vi "PicoScope3000aAdvancedTriggerSettings.vi"(0 "error in":errorcluster, 1 "handle in":i16, 3 "Trigger Conditions":T6 {"Condition Logic" items=["AND", "OR", "XOR"]}, 4 "Trigger Delay":u32, 5 "Auto Trigger (ms)":i32=1000, 6 "Channel A Trigger Properties":T3={"thresholdUpper"=0, "thresholdUpperHysteresis"=5, "thresholdLower"=0, "thresholdLowerHysteresis"=5, "Threshold Mode"=0, "Direction"=2, "Available"=FALSE} {"Direction" items=["Above / Inside", "Below / Outside", "Rising / Enter", "Falling / Exit", "Rising or Falling / Enter or Exit", "Above Lower", "Below Lower", "Rising Lower", "Falling Lower", "Positive Runt", "Negative Runt"]; "Threshold Mode" items=["Level", "Window"]}, 7 "Channel D Trigger Properties":T3={"thresholdUpper"=0, "thresholdUpperHysteresis"=0, "thresholdLower"=0, "thresholdLowerHysteresis"=0, "Threshold Mode"=0, "Direction"=2, "Available"=FALSE} {"Direction" items=["Above / Inside", "Below / Outside", "Rising / Enter", "Falling / Exit", "Rising or Falling / Enter or Exit", "Above Lower", "Below Lower", "Rising Lower", "Falling Lower", "Positive Runt", "Negative Runt"]; "Threshold Mode" items=["Level", "Window"]}, 8 "Channel B Trigger Properties":T3={"thresholdUpper"=0, "thresholdUpperHysteresis"=0, "thresholdLower"=0, "thresholdLowerHysteresis"=0, "Threshold Mode"=0, "Direction"=2, "Available"=FALSE} {"Direction" items=["Above / Inside", "Below / Outside", "Rising / Enter", "Falling / Exit", "Rising or Falling / Enter or Exit", "Above Lower", "Below Lower", "Rising Lower", "Falling Lower", "Positive Runt", "Negative Runt"]; "Threshold Mode" items=["Level", "Window"]}, 10 "Digital Port  0":T2 {"Direction Channel 7" items=["Don't Care", "Low", "High", "Rising", "Falling"]; "Direction Channel 6" items=["Don't Care", "Low", "High", "Rising", "Falling"]; "Direction Channel 5" items=["Don't Care", "Low", "High", "Rising", "Falling"]; "Direction Channel 4" items=["Don't Care", "Low", "High", "Rising", "Falling"]; "Direction Channel 3" items=["Don't Care", "Low", "High", "Rising", "Falling"]; "Direction Channel 2" items=["Don't Care", "Low", "High", "Rising", "Falling"]; "Direction Channel 1" items=["Don't Care", "Low", "High", "Rising", "Falling"]; "Direction Channel 0" items=["Don't Care", "Low", "High", "Rising", "Falling"]}, 11 "Ext. Trigger Properties":T3={"thresholdUpper"=0, "thresholdUpperHysteresis"=0, "thresholdLower"=0, "thresholdLowerHysteresis"=0, "Threshold Mode"=0, "Direction"=2, "Available"=FALSE} {"Direction" items=["Above / Inside", "Below / Outside", "Rising / Enter", "Falling / Exit", "Rising or Falling / Enter or Exit", "Above Lower", "Below Lower", "Rising Lower", "Falling Lower", "Positive Runt", "Negative Runt"]; "Threshold Mode" items=["Level", "Window"]}, 12 "Digital Port  1":T1 {"Direction Channel 15" items=["Don't Care", "Low", "High", "Rising", "Falling"]; "Direction Channel 14" items=["Don't Care", "Low", "High", "Rising", "Falling"]; "Direction Channel 13" items=["Don't Care", "Low", "High", "Rising", "Falling"]; "Direction Channel 12" items=["Don't Care", "Low", "High", "Rising", "Falling"]; "Direction Channel 11" items=["Don't Care", "Low", "High", "Rising", "Falling"]; "Direction Channel 10" items=["Don't Care", "Low", "High", "Rising", "Falling"]; "Direction Channel 9" items=["Don't Care", "Low", "High", "Rising", "Falling"]; "Direction Channel 8" items=["Don't Care", "Low", "High", "Rising", "Falling"]}, 13 "Aux. Trigger Properties":T3={"thresholdUpper"=0, "thresholdUpperHysteresis"=0, "thresholdLower"=0, "thresholdLowerHysteresis"=0, "Threshold Mode"=0, "Direction"=2, "Available"=FALSE} {"Direction" items=["Above / Inside", "Below / Outside", "Rising / Enter", "Falling / Exit", "Rising or Falling / Enter or Exit", "Above Lower", "Below Lower", "Rising Lower", "Falling Lower", "Positive Runt", "Negative Runt"]; "Threshold Mode" items=["Level", "Window"]}, 16 "Channel C Trigger Properties":T3={"thresholdUpper"=0, "thresholdUpperHysteresis"=0, "thresholdLower"=0, "thresholdLowerHysteresis"=0, "Threshold Mode"=0, "Direction"=2, "Available"=FALSE} {"Direction" items=["Above / Inside", "Below / Outside", "Rising / Enter", "Falling / Exit", "Rising or Falling / Enter or Exit", "Above Lower", "Below Lower", "Rising Lower", "Falling Lower", "Positive Runt", "Negative Runt"]; "Threshold Mode" items=["Level", "Window"]}, 18 "Pulse Width Qualifier Conditions":T5 {"Condition Logic" items=["AND", "OR", "XOR"]}, 19 "Pulse Width Qualifier Settings":T4={"Direction"=2, "Lower Limit"=0, "Upper Limit"=0, "Pulse Width Type"=0} {"Pulse Width Type" items=["None", "Less Than", "Greater Than", "In Range", "Out of Range"]; "Direction" items=["Rising"=2, "Falling"=3]}) -> (14 "error out":errorcluster, 15 "handle out":i16)   [LabVIEW 2010]
doc: "This VI is an interface for the advanced trigger features of the oscilloscope (a simple trigger can be set using PicoScope3000aSettings.vi, in which case it is not necessary to use this VI)."
uses:
  ps3000a.dll
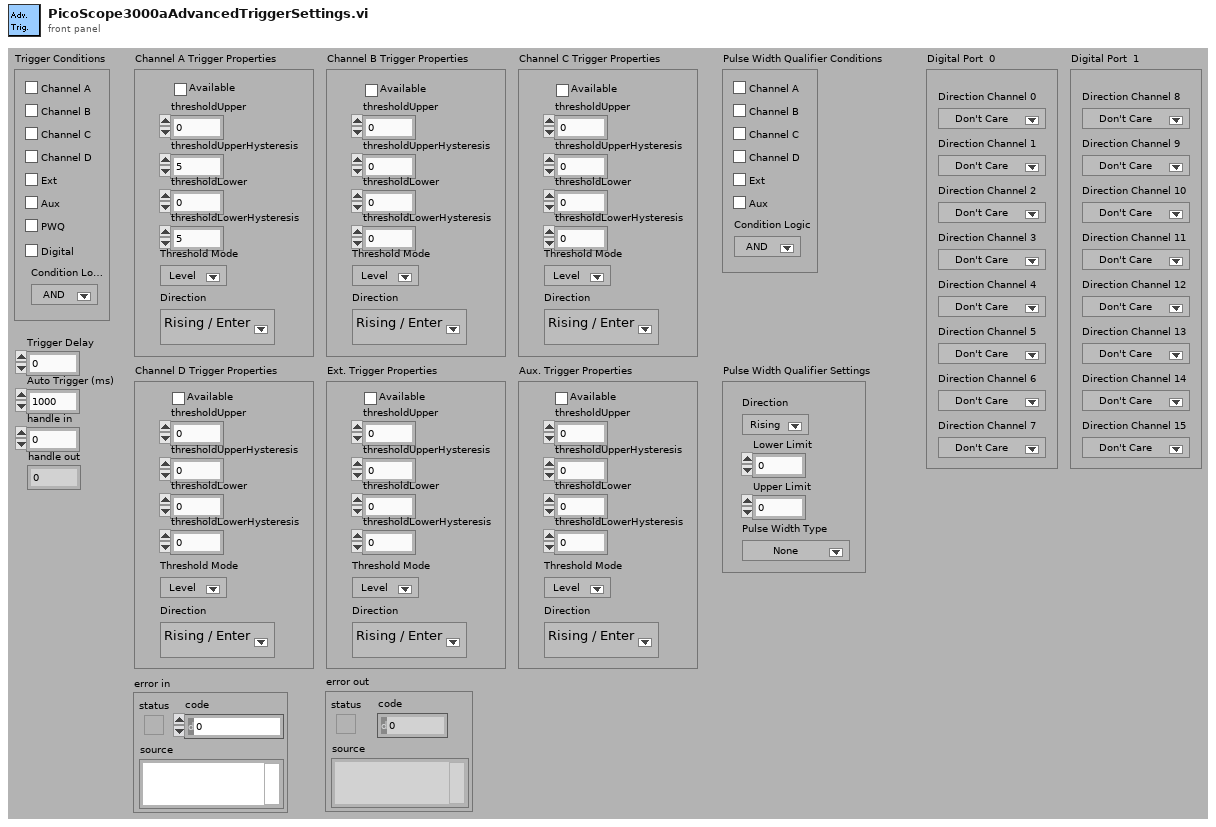
[diagram p1: front panel]
types:
  T1 = cluster{"Direction Channel 8":u16, "Direction Channel 9":u16, "Direction Channel 10":u16, "Direction Channel 11":u16, "Direction Channel 12":u16, "Direction Channel 13":u16, "Direction Channel 14":u16, "Direction Channel 15":u16}
  T2 = cluster{"Direction Channel 0":u16, "Direction Channel 1":u16, "Direction Channel 2":u16, "Direction Channel 3":u16, "Direction Channel 4":u16, "Direction Channel 5":u16, "Direction Channel 6":u16, "Direction Channel 7":u16}
  T3 = cluster{"thresholdUpper":i16, "thresholdUpperHysteresis":u16, "thresholdLower":i16, "thresholdLowerHysteresis":u16, "Threshold Mode":i32, "Direction":i32, "Available":bool}
  T4 = cluster{"Direction":u32, "Lower Limit":u32, "Upper Limit":u32, "Pulse Width Type":u32}
  T5 = cluster{"Channel A":bool, "Channel B":bool, "Channel C":bool, "Channel D":bool, "Aux":bool, "Condition Logic":u16, "Ext":bool}
  T6 = cluster{"Channel A":bool, "Channel B":bool, "Channel C":bool, "Channel D":bool, "Aux":bool, "PWQ":bool, "Condition Logic":u16, "Ext":bool, "Digital":bool}
  T7 = cluster{"thresholdUpper":i16, "thresholdUpperHysteresis":u16, "thresholdLower":i16, "thresholdLowerHysteresis":u16, "Threshold Mode":i32, "Direction":i32, "Available":bool}[]
  T8 = cluster{"[0]":u32, "[1]":u32, "[2]":u32, "[3]":u32, "[4]":u32, "[5]":u32, "[6]":u32, "[7]":u32, "[8]":u32}
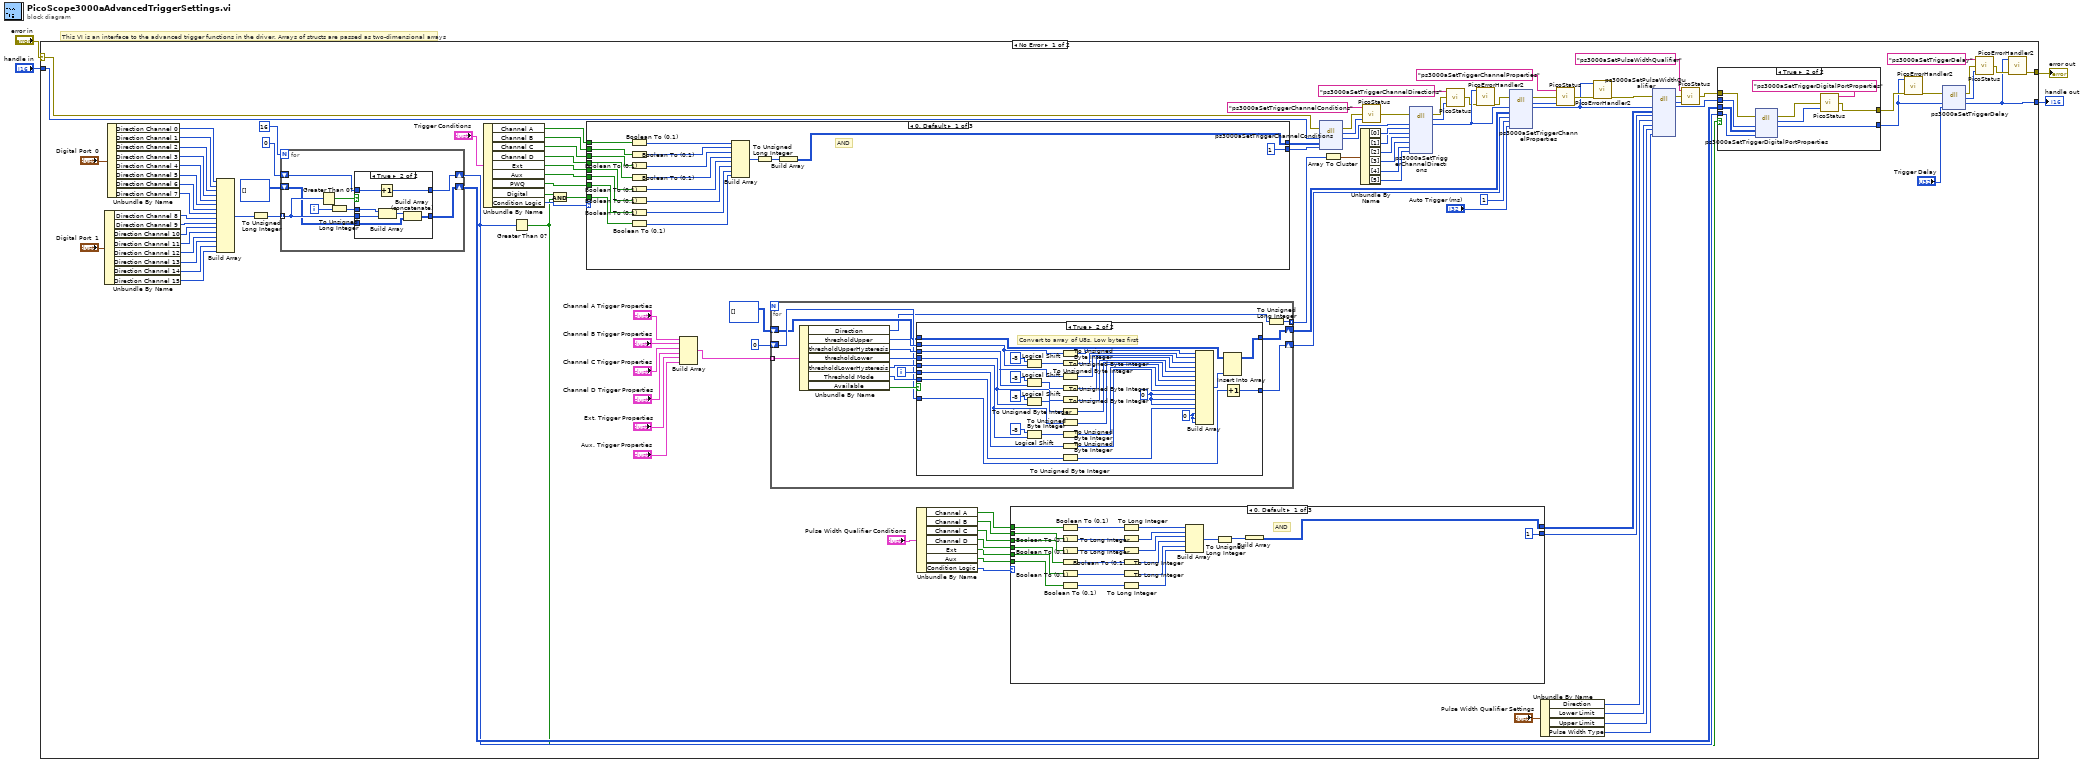
[diagram p0: block diagram]
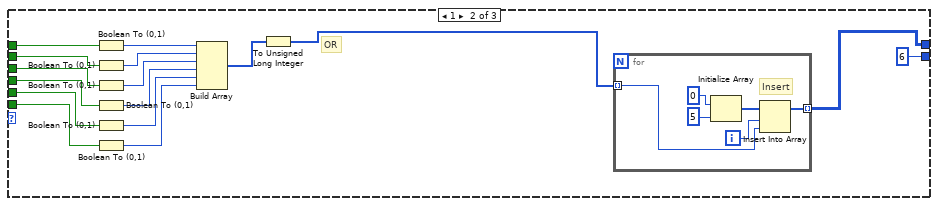
[diagram p4: hidden frame]
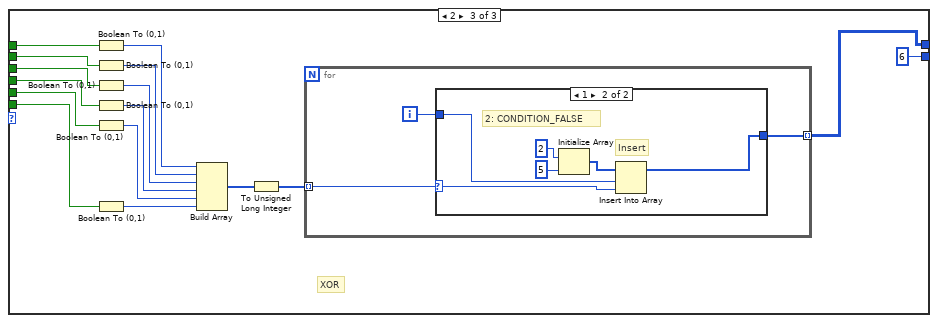
[diagram p5: hidden frame]
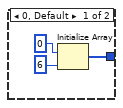
[diagram p6: hidden frame]
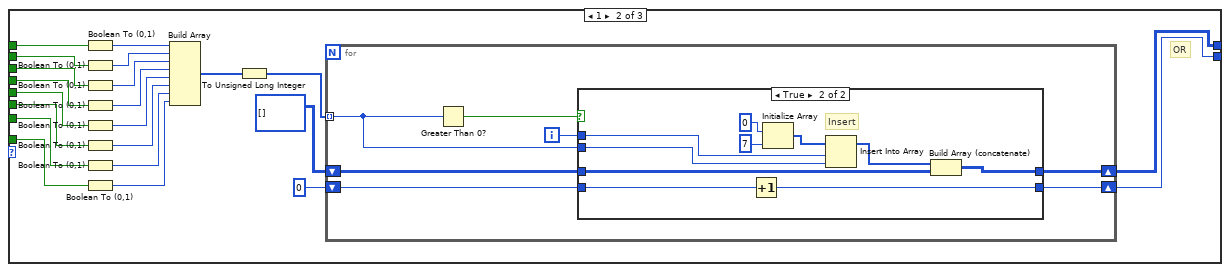
[diagram p8: hidden frame]
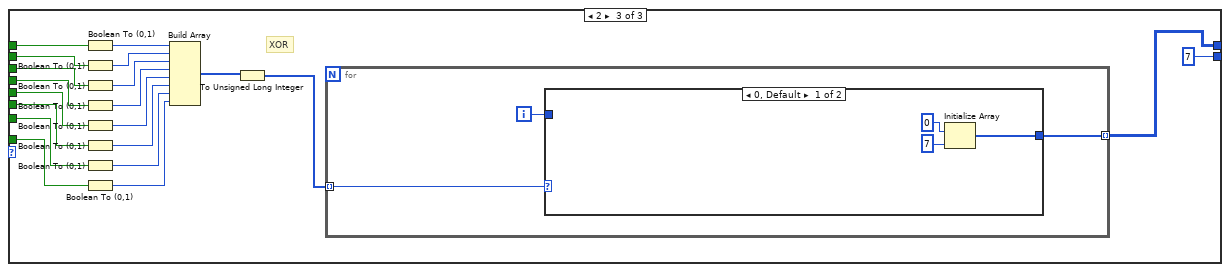
[diagram p10: hidden frame]
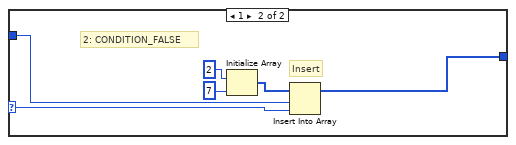
[diagram p11: hidden frame]
diagram:
  # "This VI is an interface to the advanced trigger functions in the driver. Arrays of structs are passed as two-dimensional arrays"
  n1 = case shown="No Error" "error in" {
    selector: "error in" -> [w73 w354]
    tunnel: "handle in" -> [w77 w355]
    tunnel: [w13 w355] -> w2
    tunnel: [w14 w354] -> w1
    frame No Error {
      n2 = Unbundle By Name("Digital Port  1") -> ("Direction Channel 8"=w38:u16, "Direction Channel 9"=w37:u16, "Direction Channel 10"=w36:u16, "Direction Channel 11"=w35:u16, "Direction Channel 12"=w34:u16, "Direction Channel 13"=w33:u16, "Direction Channel 14"=w32:u16, "Direction Channel 15"=w31:u16)
      n3 = Unbundle By Name("Digital Port  0") -> ("Direction Channel 0"=w50:u16, "Direction Channel 1"=w49:u16, "Direction Channel 2"=w48:u16, "Direction Channel 3"=w47:u16, "Direction Channel 4"=w46:u16, "Direction Channel 5"=w45:u16, "Direction Channel 6"=w44:u16, "Direction Channel 7"=w43:u16)
      n4 = Build Array(w50, w49, w48, w47, w46, w45, w44, w43, w38, w37, w36, w35, w34, w33, w32, w31) -> (w5:u16[])
      n5 = To Unsigned Long Integer(number=w5) -> (unsigned 32bit integer=w6:u32[])
      n6 = for {
        N: 16 -> [_]
        tunnel: w6 -> [w131] mode=indexing
        shift-right: [w130] -> w26
        shift-left: u32[][] [] -> [w129]
        shift-right: [w128] -> w23
        shift-left: i16 0 -> [w127]
        i -> [w125]
        n7 = Greater Than 0?(x=w131) -> (x > 0?=w132:bool)
        n8 = To Unsigned Long Integer(number=w125) -> (unsigned 32bit integer=w126:u32)
        n9 = case shown="True" w132 {
          tunnel: w126 -> [_ w141]
          tunnel: w131 -> [_ w140]
          tunnel: [w134 w138] -> w130
          tunnel: w129 -> [w134 w137]
          tunnel: [w133 w136] -> w128
          tunnel: w127 -> [w133 w135]
          frame False {
          }
          frame True {
            n10 = Increment(x=w135) -> (x+1=w136:i16)
            n11 = Build Array(w141, w140) -> (w139:u32[])
            n12 = Build Array (concatenate)(w139, w137) -> (w138:u32[][])
          }
        }
      }
      n13 = Unbundle By Name("Trigger Conditions") -> ("Channel A"=w57:bool, "Channel B"=w56:bool, "Channel C"=w55:bool, "Channel D"=w54:bool, "Ext"=w53:bool, "Aux"=w52:bool, "PWQ"=w51:bool, "Digital"=w25:bool, "Condition Logic"=w58:u16)
      n14 = Greater Than 0?(x=w23) -> (x > 0?=w22:bool)
      n15 = And(x=w25, y=w22) -> (x .and. y?=w24:bool)
      n16 = case shown="0, Default" w58 {
        tunnel: [w280 w295 w334] -> w110
        tunnel: [i16 1 w293 i16 7] -> w109
        tunnel: w57 -> [w278 w290 w331]
        tunnel: w56 -> [w277 w289 w330]
        tunnel: w55 -> [w276 w288 w329]
        tunnel: w54 -> [w275 w287 w328]
        tunnel: w53 -> [w274 w286 w327]
        tunnel: w52 -> [w273 w285 w326]
        tunnel: w51 -> [w272 w284 w325]
        tunnel: w24 -> [w271 w283 w324]
        frame 0, Default {
          # "AND"
          n17 = Boolean To (0,1)(Boolean=w278) -> (0, 1=w270:i16)
          n18 = Boolean To (0,1)(Boolean=w277) -> (0, 1=w269:i16)
          n19 = Boolean To (0,1)(Boolean=w276) -> (0, 1=w263:i16)
          n20 = Boolean To (0,1)(Boolean=w275) -> (0, 1=w264:i16)
          n21 = Boolean To (0,1)(Boolean=w274) -> (0, 1=w265:i16)
          n22 = Boolean To (0,1)(Boolean=w273) -> (0, 1=w266:i16)
          n23 = Boolean To (0,1)(Boolean=w272) -> (0, 1=w267:i16)
          n24 = Boolean To (0,1)(Boolean=w271) -> (0, 1=w268:i16)
          n25 = Build Array(w270, w269, w263, w264, w265, w266, w267, w268) -> (w262:i16[])
          n26 = To Unsigned Long Integer(number=w262) -> (unsigned 32bit integer=w261:u32[])
          n27 = Build Array(w261) -> (w280:u32[][])
        }
        frame 1 {
          # "OR"
          n28 = Boolean To (0,1)(Boolean=w290) -> (0, 1=w296:i16)
          n29 = Boolean To (0,1)(Boolean=w289) -> (0, 1=w297:i16)
          n30 = Boolean To (0,1)(Boolean=w288) -> (0, 1=w298:i16)
          n31 = Boolean To (0,1)(Boolean=w287) -> (0, 1=w299:i16)
          n32 = Boolean To (0,1)(Boolean=w286) -> (0, 1=w300:i16)
          n33 = Boolean To (0,1)(Boolean=w285) -> (0, 1=w301:i16)
          n34 = Boolean To (0,1)(Boolean=w284) -> (0, 1=w302:i16)
          n35 = Boolean To (0,1)(Boolean=w283) -> (0, 1=w291:i16)
          n36 = Build Array(w296, w297, w298, w299, w300, w301, w302, w291) -> (w282:i16[])
          n37 = To Unsigned Long Integer(number=w282) -> (unsigned 32bit integer=w281:u32[])
          n38 = for {
            tunnel: w281 -> [w306] mode=indexing
            shift-right: [w305] -> w295
            shift-left: u32[][] [] -> [w309]
            shift-right: [w303] -> w293
            shift-left: i16 0 -> [w304]
            i -> [w308]
            n39 = Greater Than 0?(x=w306) -> (x > 0?=w307:bool)
            n40 = case shown="True" w307 {
              tunnel: w309 -> [w311 w314]
              tunnel: w308 -> [_ w318]
              tunnel: w306 -> [_ w317]
              tunnel: [w311 w316] -> w305
              tunnel: w304 -> [w310 w313]
              tunnel: [w310 w312] -> w303
              frame False {
              }
              frame True {
                # "Insert"
                n41 = Increment(x=w313) -> (x+1=w312:i16)
                n42 = Initialize Array(u32 0 ("element"), 7 ("dimension size")) -> (w319:u32[])
                n43 = Insert Into Array(array=w319, index=w318, new element=w317) -> (w315:u32[])
                n44 = Build Array (concatenate)(w315, w314) -> (w316:u32[][])
              }
            }
          }
        }
        frame 2 {
          # "XOR"
          n45 = Boolean To (0,1)(Boolean=w331) -> (0, 1=w335:i16)
          n46 = Boolean To (0,1)(Boolean=w330) -> (0, 1=w336:i16)
          n47 = Boolean To (0,1)(Boolean=w329) -> (0, 1=w337:i16)
          n48 = Boolean To (0,1)(Boolean=w328) -> (0, 1=w338:i16)
          n49 = Boolean To (0,1)(Boolean=w327) -> (0, 1=w339:i16)
          n50 = Boolean To (0,1)(Boolean=w326) -> (0, 1=w340:i16)
          n51 = Boolean To (0,1)(Boolean=w325) -> (0, 1=w341:i16)
          n52 = Boolean To (0,1)(Boolean=w324) -> (0, 1=w332:i16)
          n53 = Build Array(w335, w336, w337, w338, w339, w340, w341, w332) -> (w323:i16[])
          n54 = To Unsigned Long Integer(number=w323) -> (unsigned 32bit integer=w322:u32[])
          n55 = for {
            tunnel: w322 -> [w342] mode=indexing
            tunnel: [w344] -> w334 mode=indexing
            i -> [w343]
            n56 = case shown="0, Default" w342 {
              selector: w342 -> [_ w349]
              tunnel: [w345 w350] -> w344
              tunnel: w343 -> [_ w348]
              frame 0, Default {
                n57 = Initialize Array(u32 0 ("element"), 7 ("dimension size")) -> (w345:u32[])
              }
              frame 1 {
                # "2: CONDITION_FALSE"
                # "Insert"
                n58 = Initialize Array(u32 2 ("element"), 7 ("dimension size")) -> (w351:u32[])
                n59 = Insert Into Array(array=w351, index=w348, new element=w349) -> (w350:u32[])
              }
            }
          }
        }
      }
      n60 = Build Array("Channel A Trigger Properties", "Channel B Trigger Properties", "Channel C Trigger Properties", "Channel D Trigger Properties", "Ext. Trigger Properties", "Aux. Trigger Properties") -> (w107:T7)
      n61 = for {
        tunnel: w107 -> [w222] mode=indexing
        tunnel: [w215] -> w106 mode=indexing
        shift-right: [w219] -> w61
        shift-left: i16 0 -> [w218]
        shift-right: [w216] -> w59
        shift-left: u8[][] [] -> [w217]
        i -> [w220]
        n62 = Unbundle By Name(w222) -> ("Direction"=w214:i32, "thresholdUpper"=w227:i16, "thresholdUpperHysteresis"=w226:u16, "thresholdLower"=w225:i16, "thresholdLowerHysteresis"=w224:u16, "Threshold Mode"=w223:i32, "Available"=w221:bool)
        n63 = case shown="True" w221 {
          tunnel: w227 -> [_ w259]
          tunnel: w226 -> [_ w251]
          tunnel: w225 -> [_ w250]
          tunnel: w224 -> [_ w249]
          tunnel: w223 -> [_ w240]
          tunnel: w220 -> [_ w235]
          tunnel: [w229 w234] -> w219
          tunnel: w218 -> [w229 w233]
          tunnel: [w228 w231] -> w216
          tunnel: w217 -> [w228 w230]
          frame False {
          }
          frame True {
            w238 = u8 0 ("element")
            w239 = u8 0 ("element")
            # "Convert to array of U8s, Low bytes first"
            n64 = Logical Shift(y=i16 -8, x=w259) -> (x << y=w258:i16)
            n65 = Logical Shift(y=i16 -8, x=w251) -> (x << y=w257:u16)
            n66 = Logical Shift(y=i16 -8, x=w250) -> (x << y=w254:i16)
            n67 = Logical Shift(y=i16 -8, x=w249) -> (x << y=w253:u16)
            n68 = To Unsigned Byte Integer(number=w259) -> (unsigned 8bit integer=w248:u8)
            n69 = To Unsigned Byte Integer(number=w258) -> (unsigned 8bit integer=w247:u8)
            n70 = To Unsigned Byte Integer(number=w251) -> (unsigned 8bit integer=w246:u8)
            n71 = To Unsigned Byte Integer(number=w257) -> (unsigned 8bit integer=w245:u8)
            n72 = To Unsigned Byte Integer(number=w250) -> (unsigned 8bit integer=w244:u8)
            n73 = To Unsigned Byte Integer(number=w254) -> (unsigned 8bit integer=w243:u8)
            n74 = To Unsigned Byte Integer(number=w249) -> (unsigned 8bit integer=w242:u8)
            n75 = To Unsigned Byte Integer(number=w253) -> (unsigned 8bit integer=w241:u8)
            n76 = To Unsigned Byte Integer(number=w235) -> (unsigned 8bit integer=w236:u8)
            n77 = To Unsigned Byte Integer(number=w240) -> (unsigned 8bit integer=w237:u8)
            n78 = Build Array(w248, w247, w246, w245, w244, w243, w242, w241, w236, w239, w239, w239, w237, w238, w238, w238) -> (w232:u8[])
            n79 = Insert Into Array(array=w230, new element=w232) -> (w231:u8[][])  [unwired: 2 in]
            n80 = Increment(x=w233) -> (x+1=w234:i16)
          }
        }
        n81 = To Unsigned Long Integer(number=w214) -> (unsigned 32bit integer=w215:u32)
      }
      n82 = Unbundle By Name("Pulse Width Qualifier Conditions") -> ("Channel A"=w96:bool, "Channel B"=w95:bool, "Channel C"=w94:bool, "Channel D"=w93:bool, "Ext"=w92:bool, "Aux"=w83:bool, "Condition Logic"=w84:u16)
      n83 = case shown="0, Default" w84 {
        tunnel: w96 -> [w163 w179 w201]
        tunnel: w95 -> [w157 w178 w200]
        tunnel: w94 -> [w156 w177 w199]
        tunnel: w93 -> [w155 w176 w198]
        tunnel: w92 -> [w154 w168 w190]
        tunnel: [w148 w170 w192] -> w91
        tunnel: [i16 1 i16 6 i16 6] -> w90
        tunnel: w83 -> [w145 w167 w189]
        frame 0, Default {
          # "AND"
          n84 = Boolean To (0,1)(Boolean=w163) -> (0, 1=w162:i16)
          n85 = Boolean To (0,1)(Boolean=w157) -> (0, 1=w161:i16)
          n86 = Boolean To (0,1)(Boolean=w156) -> (0, 1=w160:i16)
          n87 = Boolean To (0,1)(Boolean=w155) -> (0, 1=w159:i16)
          n88 = Boolean To (0,1)(Boolean=w154) -> (0, 1=w158:i16)
          n89 = Boolean To (0,1)(Boolean=w145) -> (0, 1=w146:i16)
          n90 = To Long Integer(number=w162) -> (32bit integer=w153:i32)
          n91 = To Long Integer(number=w161) -> (32bit integer=w152:i32)
          n92 = To Long Integer(number=w160) -> (32bit integer=w151:i32)
          n93 = To Long Integer(number=w159) -> (32bit integer=w150:i32)
          n94 = To Long Integer(number=w158) -> (32bit integer=w149:i32)
          n95 = To Long Integer(number=w146) -> (32bit integer=w144:i32)
          n96 = Build Array(w153, w152, w151, w150, w149, w144) -> (w142:i32[])
          n97 = To Unsigned Long Integer(number=w142) -> (unsigned 32bit integer=w143:u32[])
          n98 = Build Array(w143) -> (w148:u32[][])
        }
        frame 1 {
          # "OR"
          n99 = Boolean To (0,1)(Boolean=w179) -> (0, 1=w171:i16)
          n100 = Boolean To (0,1)(Boolean=w178) -> (0, 1=w172:i16)
          n101 = Boolean To (0,1)(Boolean=w177) -> (0, 1=w173:i16)
          n102 = Boolean To (0,1)(Boolean=w176) -> (0, 1=w174:i16)
          n103 = Boolean To (0,1)(Boolean=w168) -> (0, 1=w175:i16)
          n104 = Boolean To (0,1)(Boolean=w167) -> (0, 1=w166:i16)
          n105 = Build Array(w171, w172, w173, w174, w175, w166) -> (w165:i16[])
          n106 = To Unsigned Long Integer(number=w165) -> (unsigned 32bit integer=w164:u32[])
          n107 = for {
            tunnel: w164 -> [w181] mode=indexing
            tunnel: [w180] -> w170 mode=indexing
            i -> [w182]
            # "Insert"
            n108 = Initialize Array(u32 0 ("element"), 5 ("dimension size")) -> (w183:u32[])
            n109 = Insert Into Array(array=w183, index=w182, new element=w181) -> (w180:u32[])
          }
        }
        frame 2 {
          # "XOR"
          n110 = Boolean To (0,1)(Boolean=w201) -> (0, 1=w193:i16)
          n111 = Boolean To (0,1)(Boolean=w200) -> (0, 1=w194:i16)
          n112 = Boolean To (0,1)(Boolean=w199) -> (0, 1=w195:i16)
          n113 = Boolean To (0,1)(Boolean=w198) -> (0, 1=w196:i16)
          n114 = Boolean To (0,1)(Boolean=w190) -> (0, 1=w197:i16)
          n115 = Boolean To (0,1)(Boolean=w189) -> (0, 1=w188:i16)
          n116 = Build Array(w193, w194, w195, w196, w197, w188) -> (w187:i16[])
          n117 = To Unsigned Long Integer(number=w187) -> (unsigned 32bit integer=w186:u32[])
          n118 = for {
            tunnel: w186 -> [w204] mode=indexing
            tunnel: [w202] -> w192 mode=indexing
            i -> [w203]
            n119 = case shown="1" w204 {
              selector: w204 -> [_ w209]
              tunnel: [w205 w210] -> w202
              tunnel: w203 -> [_ w208]
              frame 0, Default {
                n120 = Initialize Array(u32 0 ("element"), 6 ("dimension size")) -> (w205:u32[])
              }
              frame 1 {
                # "2: CONDITION_FALSE"
                # "Insert"
                n121 = Initialize Array(u32 2 ("element"), 5 ("dimension size")) -> (w211:u32[])
                n122 = Insert Into Array(array=w211, index=w208, new element=w209) -> (w210:u32[])
              }
            }
          }
        }
      }
      n123 = dll-call lib="PS3000a.dll" fn="ps3000aSetTriggerChannelConditions" ("ps3000.dll:_ps3000_open_unit@0")(error in=w73, "handle"=w77, "conditions"=w110, "nConditions"=w109) -> (error out=w75:errorcluster, "PICO_STATUS"=w76:i32, "handle"=w112:i16)  [unwired: 4 in, 1 out]
      n124 = Array To Cluster(array=w106) -> (cluster=w105:T8)
      n125 = Unbundle By Name(w105) -> ("[0]"=w104:u32, "[1]"=w103:u32, "[2]"=w102:u32, "[3]"=w101:u32, "[4]"=w100:u32, "[5]"=w99:u32)
      n126 = call "PicoStatus.vi"("PICO STATUS"=w76, "error in"=w75, "source"="ps3000aSetTriggerChannelConditions") -> ("error out"=w72:errorcluster)
      n127 = dll-call lib="ps3000a.dll" fn="ps3000aSetTriggerChannelDirections" ("ps3000.dll:_ps3000_open_unit@0")(error in=w72, "handle"=w112, "channelA"=w104, "channelB"=w103, "channelC"=w102, "channelD"=w101, "ext"=w100, "aux"=w99) -> (error out=w70:errorcluster, "PICO_STATUS"=w71:i32, "handle"=w20:i16)  [unwired: 8 in, 1 out]
      n128 = call "PicoStatus.vi"("PICO STATUS"=w71, "error in"=w70, "source"="ps3000aSetTriggerChannelDirections") -> ("error out"=w19:errorcluster)
      n129 = call "PicoErrorHandler2.vi"("error in (no error)"=w19, "handle In"=w20) -> ("error out"=w21:errorcluster)  [unwired: 9 in]
      n130 = dll-call lib="ps3000a.dll" fn="ps3000aSetTriggerChannelProperties" ("ps3000.dll:_ps3000_open_unit@0")(error in=w21, "handle"=w20, "channelProperties"=w59, "nChannelProperties"=w61, "auxOutputEnable"=i16 1, "autoTriggerMilliseconds"="Auto Trigger (ms)") -> (error out=w68:errorcluster, "PICO_STATUS"=w69:i32, "handle"=w10:i16)  [unwired: 6 in, 1 out]
      n131 = Unbundle By Name("Pulse Width Qualifier Settings") -> ("Direction"=w88:u32, "Lower Limit"=w87:u32, "Upper Limit"=w86:u32, "Pulse Width Type"=w85:u32)
      n132 = call "PicoStatus.vi"("PICO STATUS"=w69, "error in"=w68, "source"="ps3000aSetTriggerChannelProperties") -> ("error out"=w11:errorcluster)
      n133 = call "PicoErrorHandler2.vi"("error in (no error)"=w11, "handle In"=w10) -> ("error out"=w12:errorcluster)  [unwired: 9 in]
      n134 = dll-call lib="ps3000a.dll" fn="ps3000aSetPulseWidthQualifier" ("ps3000.dll:_ps3000_open_unit@0")(error in=w12, "handle"=w10, "conditions"=w91, "nConditions"=w90, "direction"=w88, "lower"=w87, "upper"=w86, "type"=w85) -> (error out=w17:errorcluster, "PICO_STATUS"=w18:i32, "handle"=w27:i16)  [unwired: 8 in, 1 out]
      n135 = call "PicoStatus.vi"("PICO STATUS"=w18, "error in"=w17, "source"="ps3000aSetPulseWidthQualifier") -> ("error out"=w28:errorcluster)
      n136 = case shown="True" w22 {
        tunnel: w28 -> [w114 w123]
        tunnel: w27 -> [w115 w122]
        tunnel: [w115 w117] -> w8
        tunnel: w23 -> [_ w118]
        tunnel: w26 -> [_ w119]
        tunnel: [w114 w116] -> w9
        frame False {
        }
        frame True {
          n137 = dll-call lib="ps3000a.dll" fn="ps3000aSetTriggerDigitalPortProperties"(error in=w123, "handle"=w122, "digitalDirections"=w119, "nDigitalDirections"=w118) -> (error out=w121:errorcluster, "PICO_STATUS"=w120:i32, "handle"=w117:i16)  [unwired: 4 in, 1 out]
          n138 = call "PicoStatus.vi"("PICO STATUS"=w120, "error in"=w121, "source"="ps3000aSetTriggerDigitalPortProperties") -> ("error out"=w116:errorcluster)
        }
      }
      n139 = call "PicoErrorHandler2.vi"("error in (no error)"=w9, "handle In"=w8) -> ("error out"=w7:errorcluster)  [unwired: 9 in]
      n140 = dll-call lib="ps3000a.dll" fn="ps3000aSetTriggerDelay" ("ps3000.dll:_ps3000_open_unit@0")(error in=w7, "handle"=w8, "delay"="Trigger Delay") -> (error out=w66:errorcluster, "PICO_STATUS"=w67:i32, "handle"=w13:i16)  [unwired: 3 in, 1 out]
      n141 = call "PicoStatus.vi"("PICO STATUS"=w67, "error in"=w66, "source"="ps3000aSetTriggerDelay") -> ("error out"=w15:errorcluster)
      n142 = call "PicoErrorHandler2.vi"("error in (no error)"=w15, "handle In"=w13) -> ("error out"=w14:errorcluster)  [unwired: 9 in]
    }
    frame Error {
    }
  }
  "handle out" <- w2
  "error out" <- w1
